vi "添加产品类型.vi"(0 "Type":string) -> ()   [LabVIEW 2013]
uses:
  <vilib>/Utility/error.llb/whitespace.ctl
panel:
  out "Result":string caption="结果"
  out "error out 2":errorcluster caption="错误输出"
  out "error out":errorcluster
  out "EOF":bool
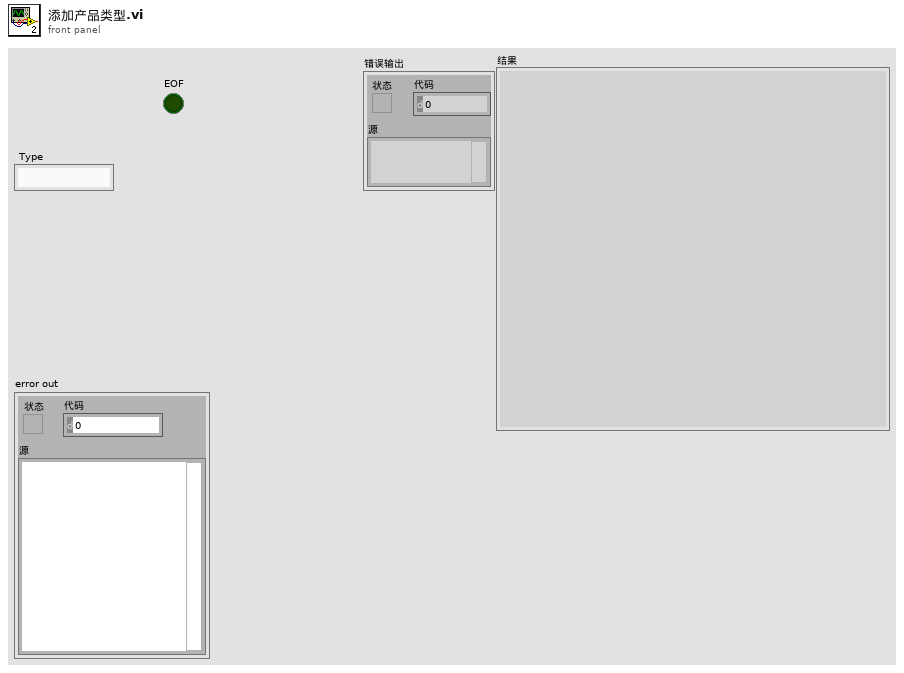
[diagram p1: front panel]
types:
  T1 = typedef "whitespace.ctl" = u16
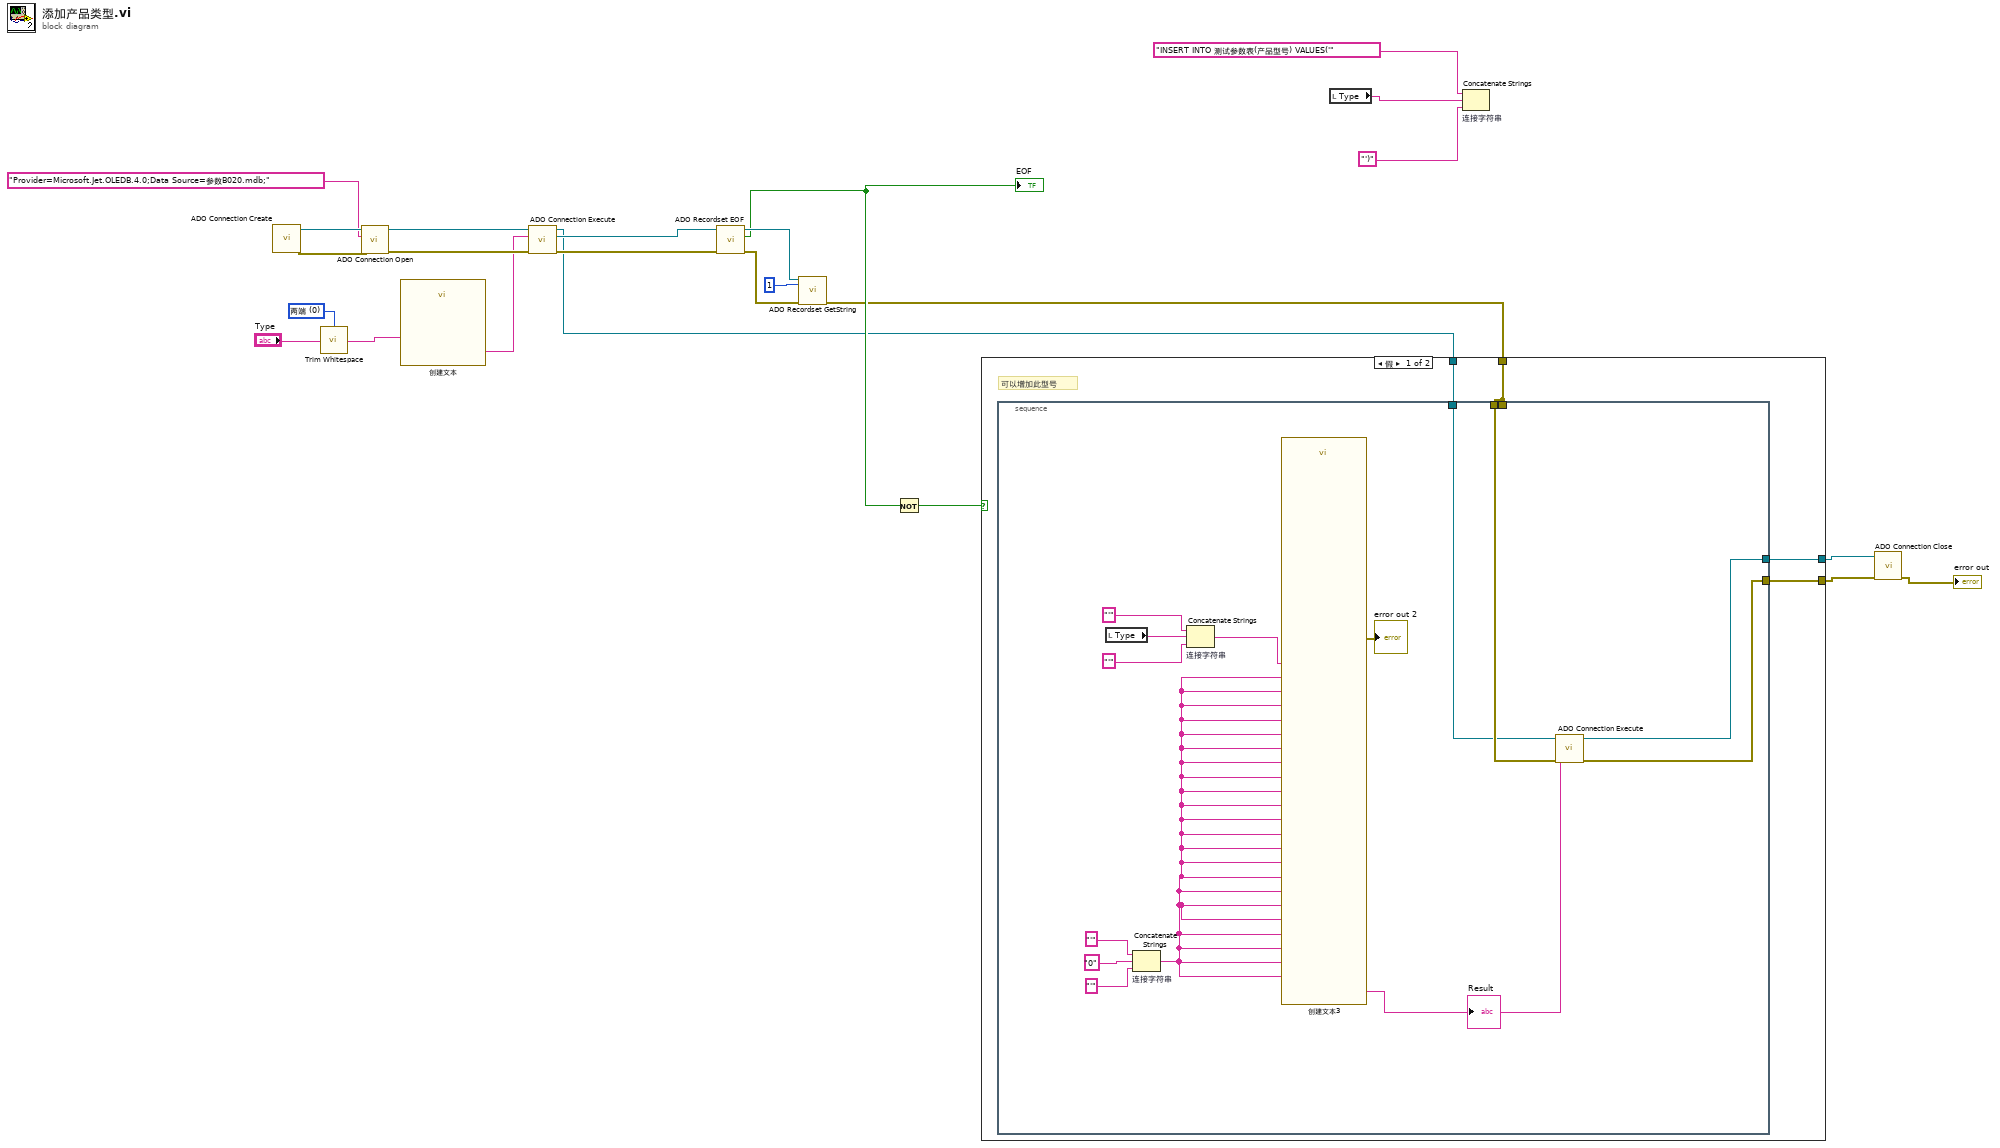
[diagram p0: block diagram]
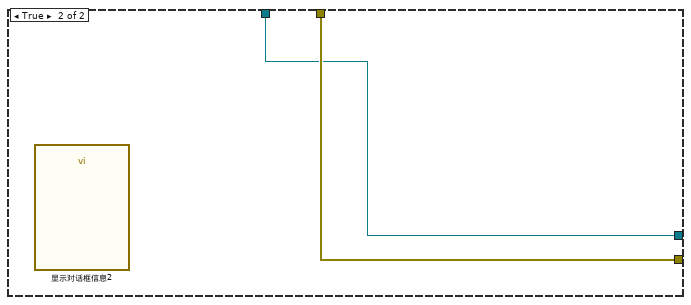
[diagram p2: hidden frame]
diagram:
  w13 = T1 0 items=["两端", "字符串首端", "字符串末端"] ("location (both)")
  n1 = call "ADO Connection Create.vi"() -> ("error out"=w23:errorcluster, "ADODB._Connection Out"=w22:refnum<k7>)  [unwired: 10 in]
  n2 = call <vilib>:"Trim Whitespace.vi"("string"="Type", "location (both)"=w13) -> ("trimmed string"=w14:string)
  n3 = call "ADO Connection Open.vi"("error in (no error)"=w23, "ConnectionString"="Provider=Microsoft.Jet.OLEDB.4.0;Data Source=参数B020.mdb;", "ADODB._Connection In"=w22) -> ("error out"=w20:errorcluster, "ADODB._Connection Out"=w16:refnum<k7>)  [unwired: 7 in]
  n4 = call "创建文本"("产品型号"=w14) -> ("Result"=w19:string)  [unwired: 13 in, 1 out]
  n5 = call "ADO Connection Execute.vi"("error in (no error)"=w20, "CommandText"=w19, "ADODB._Connection In"=w16) -> ("error out"=w24:errorcluster, "RecordSet"=w17:refnum<k7>, "ADODB._Connection Out"=w7:refnum<k7>)  [unwired: 6 in]
  n6 = call "ADO Recordset EOF.vi"("error in (no error)"=w24, "ADODB._Recordset In"=w17) -> ("error out"=w11:errorcluster, "EOF"=w10:bool, "ADODB._Recordset Out"=w12:refnum<k7>)  [unwired: 7 in]
  "EOF" <- w10
  n7 = call "ADO Recordset GetString.vi"("ADODB._Recordset"=w12, "NumRows"=1, "error in (no error)"=w11) -> ("error out"=w6:errorcluster)  [unwired: 14 in, 2 out]
  n8 = Not(x=w10) -> (.not. x?=w8:bool)
  n9 = case shown="假" w8 {
    tunnel: w7 -> [w28 w43]
    tunnel: w6 -> [w25 w44]
    tunnel: [w26 w44] -> w5
    tunnel: [w27 w43] -> w4
    frame False {
      # "可以增加此型号"
      n10 = stacked-sequence {
        tunnel: w28 -> [w33]
        tunnel: w25 -> [_]
        tunnel: [w36] -> w27
        tunnel: [w35] -> w26
        tunnel: w25 -> [w34]
        frame #0 {
          n11 = local read "Type"() -> (w41:string)
          n12 = Concatenate Strings "连接字符串"("'" ("字符串"), "0" ("字符串"), "'" ("字符串")) -> (w30:string)
          n13 = Concatenate Strings "连接字符串"("'" ("字符串"), w41, "'" ("字符串")) -> (w32:string)
          n14 = call "创建文本3"("产品型号"=w32, "区域最小位移1"=w30, "区域最大位移1"=w30, "区域最小压力1"=w30, "区域最大压力1"=w30, "最小压入位移1"=w30, "最大压入位移1"=w30, "监控点最小压力1"=w30, "监控点最大压力1"=w30, "位移监控点1"=w30, "区域最小位移2"=w30, "区域最大位移2"=w30, "区域最小压力2"=w30, "区域最大压力2"=w30, "最小压入位移2"=w30, "最大压入位移2"=w30, "监控点最小压力2"=w30, "监控点最大压力2"=w30, "位移监控点2"=w30, "伺服1快进位置设置"=w30, "伺服1快进速度设置"=w30, "伺服1慢进位置设置"=w30, "伺服1慢进速度设置"=w30) -> ("Result"=w31:string, "error out"=→"error out 2":errorcluster)  [unwired: 3 in]
          "Result" <- w31
          n15 = call "ADO Connection Execute.vi"("error in (no error)"=w34, "CommandText"=w31, "ADODB._Connection In"=w33) -> ("error out"=w35:errorcluster, "ADODB._Connection Out"=w36:refnum<k7>)  [unwired: 6 in, 1 out]
        }
      }
    }
    frame True {
      n16 = call "显示对话框信息2"() -> ()  [unwired: 10 in, 2 out]
    }
  }
  n17 = local read "Type"() -> (w2:string)
  n18 = Concatenate Strings "连接字符串"("INSERT INTO 测试参数表(产品型号) VALUES('" ("Result"), w2, "')" ("字符串")) -> ()  [unwired: 1 out]
  n19 = call "ADO Connection Close.vi"("error in (no error)"=w5, "ADODB._Connection In"=w4) -> ("error out"=→"error out":errorcluster)  [unwired: 8 in, 1 out]
